vi "delta 0.1.vi"() -> ()   [LabVIEW 2019]
uses:
  lib/Keithley 622x/Configure/Format/Typedefs/KE622x -- Results Format.ctl
  lib/Keithley 622x/Configure/Format/Typedefs/KE622x -- Optional Meas Elements.ctl
  lib/Keithley 622x/Configure/Delta PDelta DCon Modes/Typedefs/KE622x -- Delta Mode Params.ctl
  lib/Keithley 622x/Configure/Delta PDelta DCon Modes/Low Level/Typedefs/KE622x -- Delta PDelta Mode High Level.ctl
  lib/Keithley 622x/Configure/Delta PDelta DCon Modes/Low Level/Typedefs/KE622x -- Delta PDelta Mode Low Level.ctl
  lib/Keithley 622x/Configure/Delta PDelta DCon Modes/Low Level/Typedefs/KE622x -- Delta DCon Mode Delay.ctl
  lib/Keithley 622x/Configure/Delta PDelta DCon Modes/Low Level/Typedefs/KE622x -- Delta PDelta Mode Num Cycles Mode.ctl
  lib/Keithley 622x/Configure/Delta PDelta DCon Modes/Low Level/Typedefs/KE622x -- Delta PDelta Mode Num Cycles.ctl
  lib/Keithley 622x/Configure/2182 -A/Low Level/Typedefs/KE2182 -- Voltage Ranges.ctl
  lib/Keithley 622x/Configure/2182 -A/Low Level/Typedefs/KE2182 -- Filter Type.ctl
  lib/Keithley 622x/Configure/2182 -A/Low Level/Typedefs/KE2182 -- Filter Count.ctl
  lib/Keithley 622x/Configure/2182 -A/Low Level/Typedefs/KE2182 -- Filter Window.ctl
  lib/Keithley 622x/Configure/2182 -A/Low Level/Typedefs/KE2182 -- NPLCs.ctl
  lib/Keithley 622x/Configure/Units/Typedefs/KE622x -- Voltage Meas Units.ctl
  KE7001.LLB/Keith 7001 Open/Close Chan.vi
  <vilib>/Utility/file.llb/Write Delimited Spreadsheet (DBL).vi
  lib/Keithley 622x/Keithley 622x.lvlib
panel:
  in  "Meas Units":T1=enum."Ohms"
  out "XY图":cluster{dbl[], dbl[]}(graph)
  in  "file path (dialog if empty)":path caption="文件路径 （空时为对话框）"
  in  "622x Resource":refnum<visa-resource-name>
  in  "Check For SCPI Errors? (T)":bool=TRUE
  in  "2182/2182A Delta Mode Meas Params":T7={"Auto Range?"=TRUE, "Man / Selected\nRange"=enum."10mV", "Enable Digital\nFilter?"=FALSE, "Filter Type"=enum."Moving", "Filter Count"=10, "Filter\nWindow (%)"=0.01, "Enable Analog\nFilter?"=FALSE, "NPLCs"=5} {"Filter\nWindow (%)" min=0.0 max=10.0 step=0.01 format="%.2f"; "Filter Count" min=1 max=100; "NPLCs" min=1 max=10}
  in  "622x Delta Meas Mode Params":T8={"High Level (A)"=0.001, "Low Level (A)"=-0.001, "Delay (s)"=0.002, "Num Cycles Mode"=enum."Finite Count", "Finite Count"=10, "Abort On\nCompliance?"=FALSE, "Cold Swithing\nMode Enabled?"=FALSE} {"Finite Count" min=2 max=65536; "Low Level (A)" min=-0.105 max=0.0 format="%.3p"; "High Level (A)" min=0.0 max=0.105 format="%.3p"; "Delay (s)" min=0.001 max=9999.999 format="%.3f"}
  in  "Meas Timeout\n(msecs)":u32=20000
  out "Execution Time\n(secs)":dbl
  out "Meas\nTimeout?":bool
  in  "Meas Elements To Return":T14={"Timstamp?"=TRUE, "Reading Num?"=TRUE, "Source Value?"=TRUE, "Compliance?"=TRUE, "Average Voltage?"=TRUE}
  in  "Results Format":T15={"Results Format"=enum."Single Prec Bin", "Bin Byte Order"=enum."Swapped"}
  in  "Instrument Type":i32(ring)=3 items=["PPMS", "VersaLab", "DynaCool", "SVSM"]
  # "*** NOTE:  \"Average Voltage\"\nis only available for Differential\nConductance measurements."
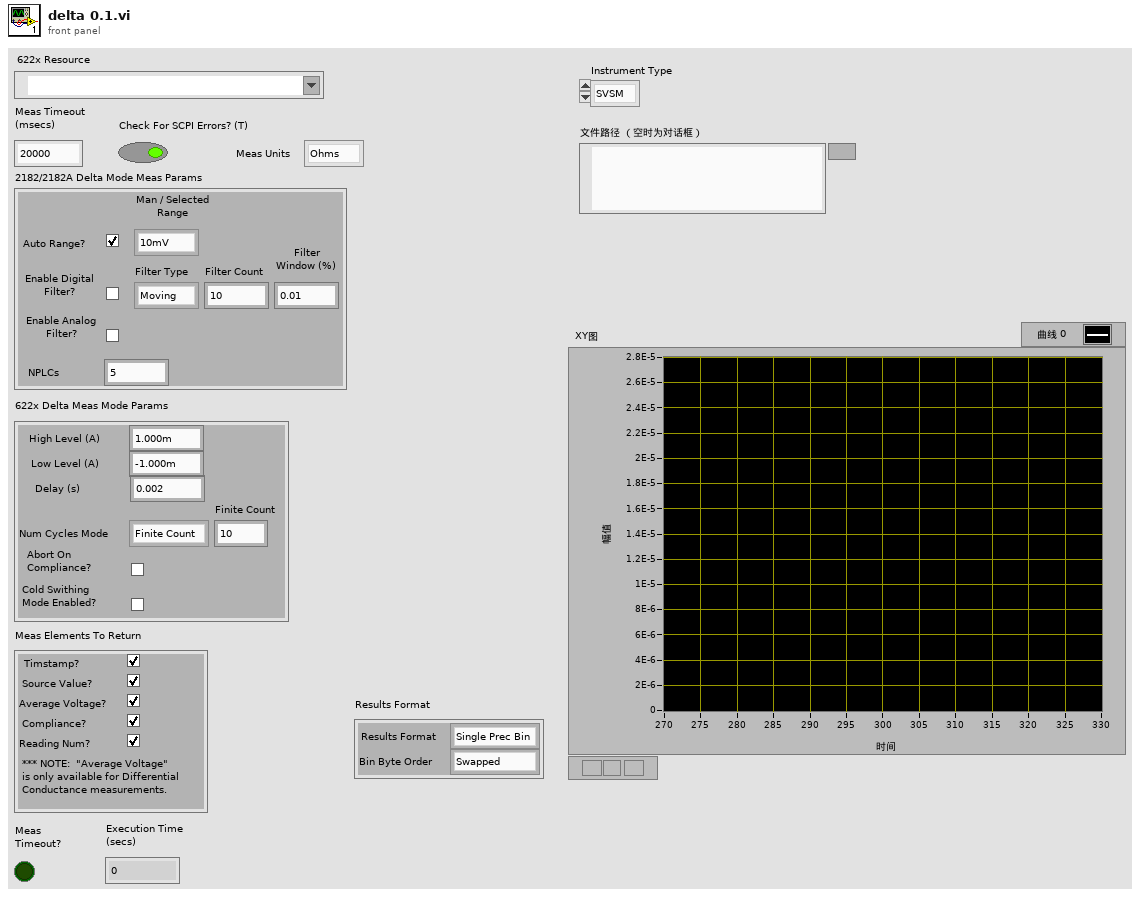
[diagram p1: front panel]
types:
  T1 = typedef "Keithley 622x.lvlib/KE622x -- Voltage Meas Units.ctl" = enum16{"Volts", "Ohms", "Watts", "Siemens"}
  T2 = typedef "Keithley 622x.lvlib/KE2182 -- Voltage Ranges.ctl" = enum16{"10mV", "100mV", "1V", "10V", "100V"}
  T3 = typedef "Keithley 622x.lvlib/KE2182 -- Filter Type.ctl" = enum16{"Moving", "Repeat"}
  T4 = typedef "Keithley 622x.lvlib/KE2182 -- Filter Count.ctl" = u32
  T5 = typedef "Keithley 622x.lvlib/KE2182 -- Filter Window.ctl" = dbl
  T6 = typedef "Keithley 622x.lvlib/KE2182 -- NPLCs.ctl" = u32
  T7 = cluster{"Auto Range?":bool, "Man / Selected\nRange":T2, "Enable Digital\nFilter?":bool, "Filter Type":T3, "Filter Count":T4, "Filter\nWindow (%)":T5, "Enable Analog\nFilter?":bool, "NPLCs":T6}
  T8 = typedef "Keithley 622x.lvlib/KE622x -- Delta Mode Params.ctl" = cluster{"High Level (A)":T9, "Low Level (A)":T10, "Delay (s)":T11, "Num Cycles Mode":T12, "Finite Count":T13, "Abort On\nCompliance?":bool, "Cold Swithing\nMode Enabled?":bool}
  T9 = typedef "Keithley 622x.lvlib/KE622x -- Delta PDelta Mode High Level.ctl" = dbl
  T10 = typedef "Keithley 622x.lvlib/KE622x -- Delta PDelta Mode Low Level.ctl" = dbl
  T11 = typedef "Keithley 622x.lvlib/KE622x -- Delta DCon Mode Delay.ctl" = dbl
  T12 = typedef "Keithley 622x.lvlib/KE622x -- Delta PDelta Mode Num Cycles Mode.ctl" = enum16{"Finite Count", "Infinite"}
  T13 = typedef "Keithley 622x.lvlib/KE622x -- Delta PDelta Mode Num Cycles.ctl" = u32
  T14 = typedef "Keithley 622x.lvlib/KE622x -- Optional Meas Elements.ctl" = cluster{"Timstamp?":bool, "Reading Num?":bool, "Source Value?":bool, "Compliance?":bool, "Average Voltage?":bool}
  T15 = typedef "Keithley 622x.lvlib/KE622x -- Results Format.ctl" = cluster{"Results Format":enum16{"ASCII", "Single Prec Bin", "Double Prec Bin"}, "Bin Byte Order":enum16{"Normal", "Swapped"}}
  T16 = enum16{"open", "replace", "create", "open or create", "replace or create", "replace or create with confirmation"}
  T17 = cluster{"slot/memory":i16, "channel/row":i16, "column":i16, bool, bool}[]
  T18 = typedef "Keithley 622x.lvlib/KE622x -- Trace Buf.ctl" = cluster{"Additional Valid Arrays":T14, "Reading Num":u32[], "Timestamp (secs)":sgl[], "Source Val (A)":sgl[], "Reading":sgl[], "Average Voltage (V)":sgl[], "Compliance?":bool[]}
  T19 = cluster{"error":bool, "code":i32, "source":string}
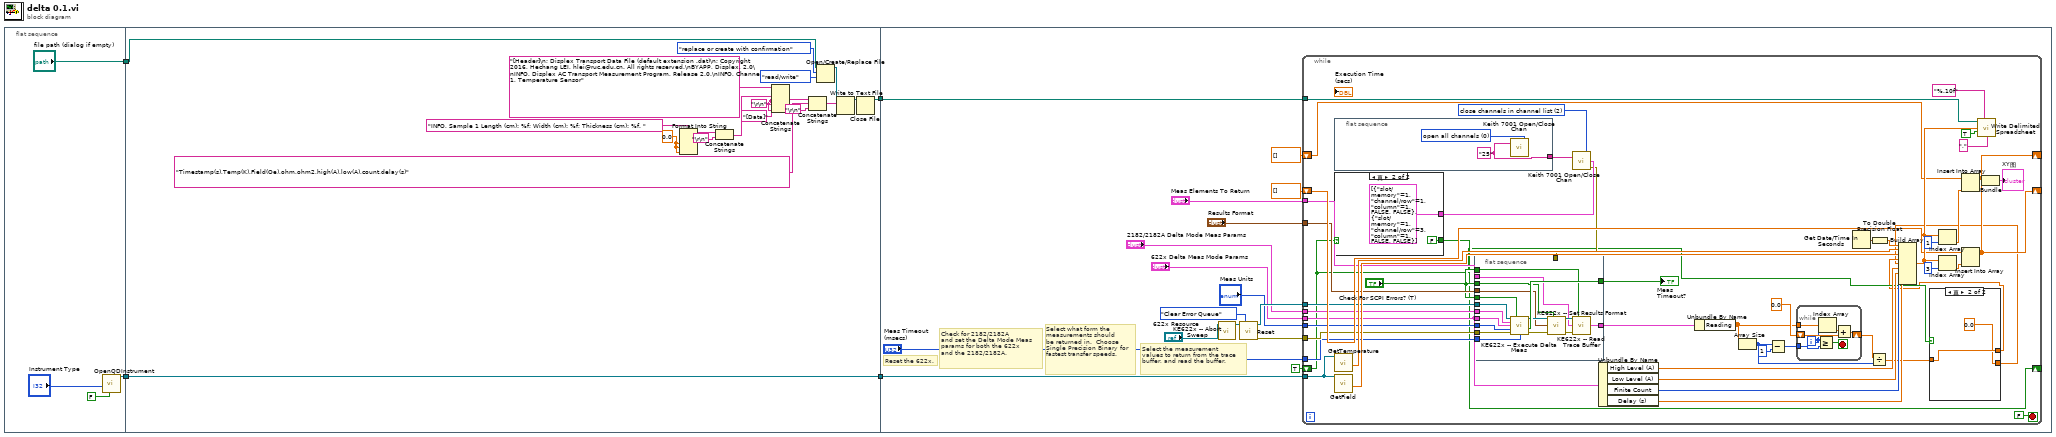
[diagram p0: block diagram]
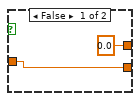
[diagram p2: hidden frame]
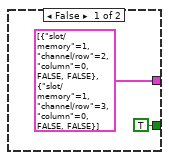
[diagram p3: hidden frame]
diagram:
  n1 = flat-sequence {
    tunnel: [w6] -> w4
    tunnel: ["file path (dialog if empty)"] -> w2
    tunnel: w4 -> [w27]
    tunnel: [w27] -> w3
    tunnel: w2 -> [w15]
    tunnel: [w10] -> w1
    tunnel: w3 -> [w43]
    tunnel: w1 -> [w34]
    frame #0 {
      n2 = call "OpenQDInstrument.vi"("Remote"=FALSE, "Instrument Type"="Instrument Type") -> ("Instrument Ref"=w6:refnum<k24>)  [unwired: 6 in, 1 out]
    }
    frame #1 {
      w22 = 0.0 ("输入 1")
      w19 = "\r\n"
      n3 = Format Into String(format string="INFO, Sample 1 Length (cm): %f; Width (cm): %f; Thickness (cm): %f. " ("string"), w22, w22, w22) -> (resulting string=w24:string)  [unwired: 2 in, 1 out]
      n4 = Concatenate Strings(w24, "\r\n") -> (w26:string)
      n5 = Concatenate Strings("[Header]\n; Displex Transport Data File (default extension .dat)\n; Copyright 2016, Hechang LEI, hlei@ruc.edu.cn. All rights reserved.\nBYAPP, Displex, 2.0\nINFO, Displex AC Transport Measurement Program, Release 2.0.\nINFO, Channel 1, Temperature Sensor" ("string"), w19, w26, w19, "[Data]" ("string"), w19) -> (w25:string)
      n6 = Concatenate Strings(w25, "Timestamp(s),Temp(K),Field(Oe),ohm,ohm2,high(A),low(A),count,delay(s)" ("字符串"), "\r\n") -> (w16:string)
      n7 = Open/Create/Replace File(file path (use dialog)=w15, operation (0:open)=T16."replace or create with confirmation" ("操作(0:open)"), access (0:read/write)=enum16{"read/write", "read-only", "write-only"}."read/write" ("权限(0:read/write)")) -> (refnum out=w14:refnum<file>)  [unwired: 3 in, 2 out]
      n8 = Write to Text File(file (use dialog)=w14, text=w16) -> (refnum out=w11:refnum<file>)  [unwired: 2 in, 2 out]
      n9 = Close File(refnum=w11) -> (path=w10:path)  [unwired: 1 in, 1 out]
    }
    frame #2 {
      # "Select what form the\nmeasurements should\nbe returned in.  Choose\nSingle Precision Binary for\nfastest transfer speeds."
      # "Select the measurement\nvalues to return from the trace\nbuffer, and read the buffer."
      # "Check for 2182/2182A\nand set the Delta Mode Meas\nparams for both the 622x\nand the 2182/2182A."
      # "Reset the 622x."
      n10 = call "KE622x -- Abort Sweep.vi"("Resource In"="622x Resource") -> ("Resource Out (dupl)"=w30:refnum<visa-resource-name>)  [unwired: 13 in, 1 out]
      n11 = call "Reset.vi"("VISA resource name"=w30, "Error Queue Option"=enum16{"Clear Error Queue", "Error Query"}."Clear Error Queue") -> ("VISA resource name out"=w41:refnum<visa-resource-name>, "error out"=w38:errorcluster)  [unwired: 12 in]
      n12 = while {
        tunnel: w43 -> [w92]
        tunnel: w41 -> [w60]
        tunnel: "2182/2182A Delta Mode Meas Params" -> [w59]
        tunnel: "622x Delta Meas Mode Params" -> [w58]
        tunnel: "Meas Units" -> [w57]
        tunnel: w38 -> [w56]
        tunnel: "Meas Timeout\n(msecs)" -> [w55]
        tunnel: "Meas Elements To Return" -> [w51]
        tunnel: "Results Format" -> [w53]
        tunnel: w34 -> [w82]
        shift-right: [w67] -> _
        shift-left: T11[] [] -> [w70]
        shift-right: [w68] -> _
        shift-left: T11[] [] -> [w72]
        shift-right: [w48] -> _
        shift-left: TRUE -> [w47]
        stop <- FALSE stop-if-true
        w63 = u16 2 items=["open all channels", "open channels in channel list", "close channels in channel list"] ("open/close (open all:0)")
        n13 = flat-sequence {
          tunnel: [w119] -> w62
          frame #0 {
            w120 = u16 0 items=["open all channels", "open channels in channel list", "close channels in channel list"] ("open/close (open all:0)")
            w119 = "25" ("GPIB address")
            n14 = call "Keith 7001 Open/Close Chan.vi"("GPIB address"=w119, "open/close (open all:0)"=w120) -> ()  [unwired: 2 in, 1 out]
          }
        }
        n15 = case shown="真" w47 {
          tunnel: [T17 [{"slot/memory"=1, "channel/row"=2, "column"=0, FALSE, FALSE}, {"slot/memory"=1, "channel/row"=3, "column"=0, FALSE, FALSE}] ("channel list") T17 [{"slot/memory"=1, "channel/row"=1, "column"=1, FALSE, FALSE}, {"slot/memory"=1, "channel/row"=3, "column"=1, FALSE, FALSE}] ("channel list")] -> w61
          tunnel: [TRUE FALSE] -> w48
          frame False {
          }
          frame True {
          }
        }
        n16 = call "GetTemperature.vi"("Instrument Ref In"=w92) -> ("Temperature"=w91:dbl)  [unwired: 4 in, 4 out]
        n17 = call "GetField.vi"("Instrument Ref In"=w92) -> ("Field"=w90:dbl)  [unwired: 4 in, 4 out]
        n18 = flat-sequence {
          tunnel: w60 -> [w114]
          tunnel: "Check For SCPI Errors? (T)" -> [w113]
          tunnel: w59 -> [w112]
          tunnel: w58 -> [w111]
          tunnel: w57 -> [w110]
          tunnel: w56 -> [w109]
          tunnel: w55 -> [w108]
          tunnel: [w107] -> w54
          tunnel: "Check For SCPI Errors? (T)" -> [w105]
          tunnel: w53 -> [w104]
          tunnel: "Check For SCPI Errors? (T)" -> [w101]
          tunnel: w51 -> [w100]
          tunnel: [w98] -> w50
          tunnel: w49 -> [_]
          frame #0 {
            n19 = call "KE622x -- Execute Delta Meas.vi"("Resource In"=w114, "Check For SCPI Errors? (T)"=w113, "2812 -A Params In"=w112, "Delta Mode Params In"=w111, "Meas Units"=w110, "error in (no error)"=w109, "Timeout (20000 ms)"=w108) -> ("Resource Out (dupl)"=w106:refnum<visa-resource-name>, "Timeout?"=w107:bool, "error out"=w103:errorcluster)  [unwired: 3 in, 3 out]
            n20 = call "KE622x -- Set Results Format.vi"("Resource In"=w106, "Check For SCPI Errors? (T)"=w105, "Results Format"=w104, "error in (no error)"=w103) -> ("Resource Out (dupl)"=w102:refnum<visa-resource-name>, "error out"=w99:errorcluster)  [unwired: 10 in]
            n21 = call "KE622x -- Read Trace Buffer.vi"("Resource In"=w102, "Check For SCPI Errors? (T)"=w101, "Meas Elements To Return"=w100, "error in (no error)"=w99) -> ("Trace Buf"=w98:T18)  [unwired: 9 in, 2 out]
          }
        }
        n22 = call "Keith 7001 Open/Close Chan.vi"("GPIB address"=w62, "open/close (open all:0)"=w63, "channel list"=w61) -> ("error out"=w49:T19)  [unwired: 1 in]
        n23 = Unbundle By Name(w58) -> ("High Level (A)"=w79:T9, "Low Level (A)"=w78:T10, "Finite Count"=w77:T13, "Delay (s)"=w76:T11)
        n24 = Unbundle By Name(w50) -> ("Reading"=w87:sgl[])
        n25 = Array Size(array=w87) -> (size(s)=w64:i32)
        n26 = Subtract(x=w64, y=1) -> (x-y=w85:i32)
        n27 = while {
          tunnel: w87 -> [w127]
          shift-right: [w124] -> w88
          shift-left: sgl 0.0 ("Numeric") -> [w125]
          tunnel: w85 -> [w123]
          i -> [w122]
          stop <- w121 stop-if-true
          n28 = Greater Or Equal?(x=w122, y=w123) -> (x >= y?=w121:bool)
          n29 = Index Array(array=w127, index=w122) -> (element=w126:sgl)
          n30 = Add(x=w126, y=w125) -> (x+y=w124:sgl)
        }
        n31 = Get Date/Time In Seconds() -> (seconds since 1Jan1904=w81:timestamp)
        n32 = Divide(x=w88, y=w64) -> (x/y=w46:sgl)
        n33 = To Double Precision Float(number=w81) -> (double precision float=w80:dbl)
        n34 = case shown="真" w47 {
          tunnel: w46 -> [w95 w97]
          tunnel: [sgl 0.0 w97] -> w45
          tunnel: [w95 sgl 0.0 ("Numeric")] -> w44
          frame False {
          }
          frame True {
          }
        }
        n35 = Build Array(w80, w91, w90, w45, w44, w79, w78, w77, w76) -> (w73:T11[])
        n36 = Index Array(array=w73, index=1 ("索引")) -> (element=w71:T11)
        n37 = Index Array(array=w73, index=3 ("索引")) -> (element=w69:T11)
        n38 = Insert Into Array(array=w72, new element=w71) -> (w68:T11[])  [unwired: 1 in]
        n39 = Insert Into Array(array=w70, new element=w69) -> (w67:T11[])  [unwired: 1 in]
        n40 = call-poly <vilib>:"Write Delimited Spreadsheet.vi"("file path (dialog if empty)"=w82, "format (%.3f)"="%.10f", "1D data"=w73, "append to file? (new file:F)"=TRUE, "delimiter (\\t)"="," ("delimiter (\\t)")) -> ()  [unwired: 9 in, 2 out]
        n41 = Bundle(w68, w67) -> (→"XY图":cluster{T11[], T11[]})  [unwired: 1 in]
        "Meas\nTimeout?" <- w54
      }
    }
  }
